vi "collectLT_img_old.vi"() -> (0 "cts/sec":dbl, 1 "counts":i32)   [LabVIEW 2013]
uses:
  phlib.dll
panel:
  out "index of element":i32
  out "trunc buffer":u32[](array[numeric]) format="%08x"
  out "buffer":u32[](array[numeric]) format="%08x"
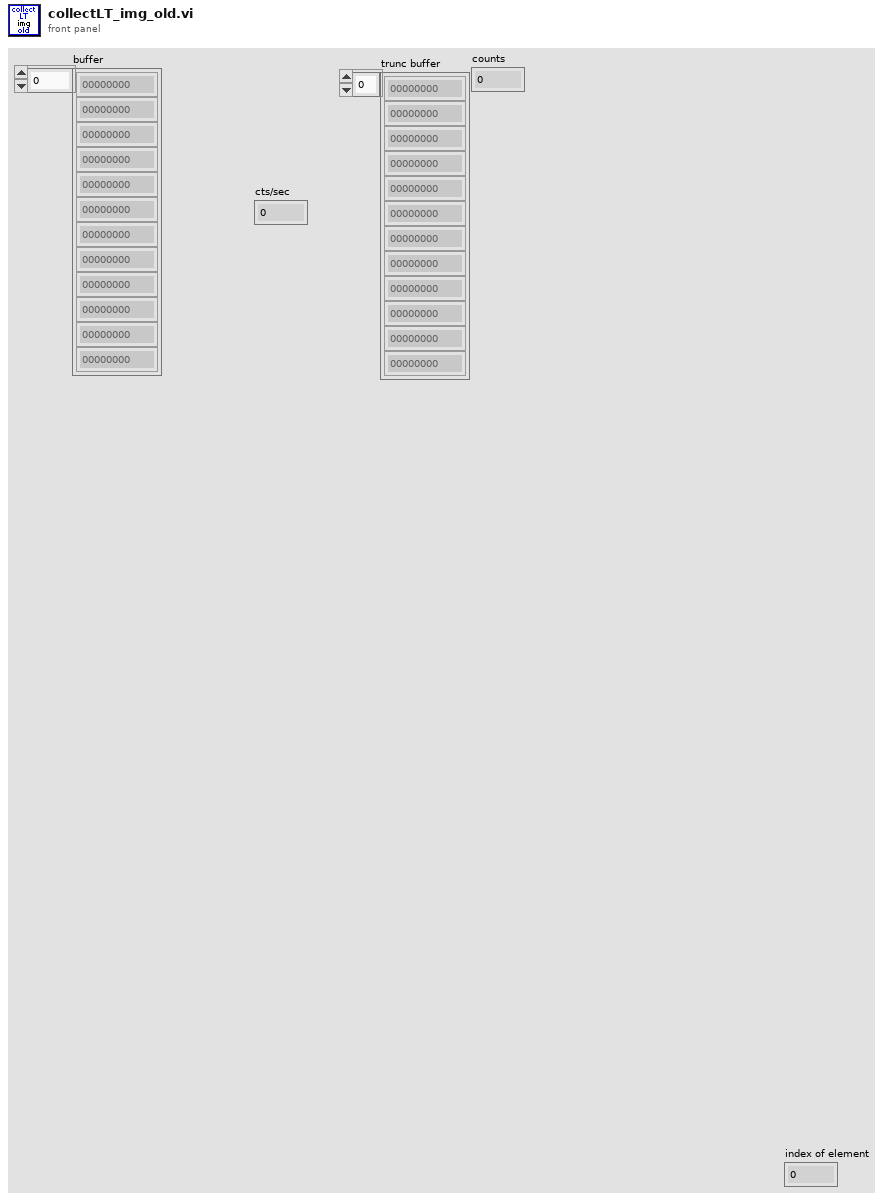
[diagram p1: front panel]
types:
  T1 = cluster{"Z_n":i32[], "devidx":i32, "initialized":bool, "acq time":i32, "Bin size":enum16{"1", "2", "4", "8", "16", "32", "64", "128"}, "# bins":u32, "sync rate":i32, "Ch0 Level":i32, "Ch1 Level":i32, "Ch0 ZeroX":i32, "Ch1 ZeroX":i32, "resolution":i32, "collect":bool, "min photons":u32, "truncate":u32}
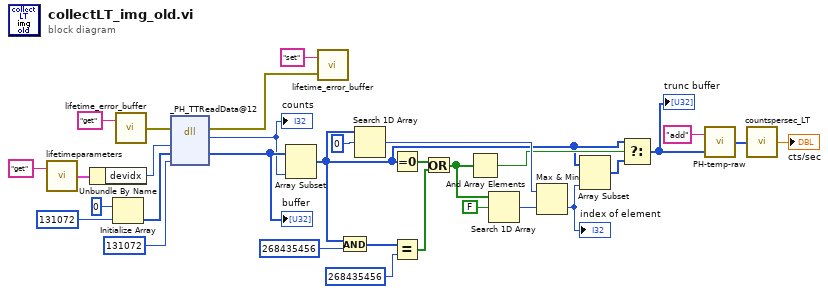
[diagram p0: block diagram]
diagram:
  n1 = call "lifetimeparameters.vi"("command"="get") -> ("Params out"=w28:T1)  [unwired: 1 in]
  n2 = Unbundle By Name(w28) -> ("devidx"=w19:i32)
  n3 = Initialize Array(u32 0, 131072 ("dimension size")) -> (w21:u32[])
  n4 = call "lifetime_error_buffer.vi"("command"="get") -> ("error out"=w30:errorcluster)  [unwired: 1 in]
  n5 = dll-call lib="phlib.dll" fn="_PH_TTReadData@12" label="PH_TTReadData"(error in=w30, "devidx"=w19, "buffer"=w21, "blocksize"=131072) -> (error out=w18:errorcluster, "return type"=w1:i32, "buffer"=w2:u32[])  [unwired: 4 in, 1 out]
  "buffer" <- w2
  "counts" <- w1
  n6 = Array Subset(array=w2, length=w1) -> (w4:u32[])  [unwired: 1 in]
  n7 = call "lifetime_error_buffer.vi"("error in"=w18, "command"="set") -> ()  [unwired: 1 out]
  n8 = And(x=w4, y=u32 268435456 ("blocksize")) -> (x .and. y?=w9:u32[])
  n9 = Search 1D Array(1D array=w4, element=u32 0) -> (index of element=w16:i32)  [unwired: 1 in]
  n10 = Equal To 0?(x=w4) -> (x = 0?=w11:bool[])
  n11 = Equal?(x=w9, y=u32 268435456 ("blocksize")) -> (x = y?=w10:bool[])
  n12 = Or(x=w11, y=w10) -> (x .or. y?=w13:bool[])
  n13 = And Array Elements(Boolean array=w13) -> (logical AND=w12:bool)
  n14 = Search 1D Array(1D array=w13, element=FALSE) -> (index of element=w17:i32)  [unwired: 1 in]
  n15 = Max & Min(x=w16, y=w17) -> (min(x,y)=w5:i32)  [unwired: 1 out]
  "index of element" <- w5
  n16 = Array Subset(array=w4, length=w5) -> (w6:u32[])  [unwired: 1 in]
  n17 = Select(t=w4, s=w12, f=w6) -> (s? t:f=w3:u32[])
  "trunc buffer" <- w3
  n18 = call "PH-temp-raw.vi"("array in"=w3, "command"="add") -> ("array out"=w22:u32[])
  n19 = call "countspersec_LT.vi"("1D PH data"=w22) -> ("Avg cts/s"=→"cts/sec":dbl)
